vi "Teardown Create.vi"(8 "Error in":errorcluster, 10 "Actor in":refnum<class "Actor.lvclass">) -> (2 "Actor out":refnum<class "Actor.lvclass">)   [LabVIEW 2020, in "jettl.lvlib" / "Actor.lvlib"]
uses:
  Actor.lvlib
  Actor/Actor.lvclass
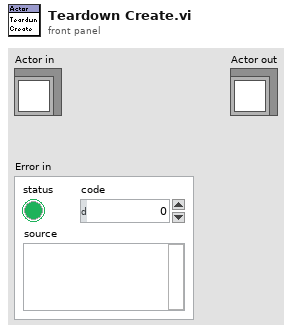
[diagram p1: front panel]
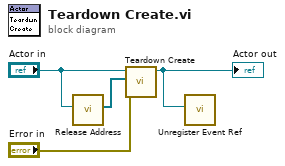
[diagram p0: block diagram]
diagram:
  n1 = call "Release Address.vi"("Actor"="Actor in") -> ("Unhandled Msgs"=w2:refnum<class "Msg.lvclass">[])  [unwired: 10 in]
  n2 = call-dynamic "Teardown Create.vi"("Error in"="Error in", "Unhandled Msgs"=w2, "Actor in"="Actor in") -> ("Actor out"=w1:refnum<class "Actor.lvclass">)  [unwired: 8 in]
  "Actor out" <- w1
  n3 = call "Unregister Event Ref.vi"("Actor"=w1) -> ()  [unwired: 11 in]
